vi "Parse Version String.vi"(11 "Version String":string) -> (3 "Version":T1)   [LabVIEW 2021, in "CIFPluginManager.lvclass"]
uses:
  CIFCore/Common/Typedef/Version.ctl
  <vilib>/regexp/Match Regular Expression.xnode
  CIFPluginManager.lvclass
  CIFPluginManager.lvclass/CIFPluginManager.ctl
  CIFCore/Common/CIFCoreCommon.lvlib
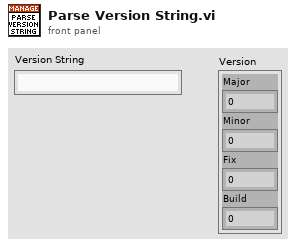
[diagram p1: front panel]
types:
  T1 = typedef "CIFCoreCommon.lvlib/Version.ctl" = cluster{"Major":i32, "Minor":i32, "Fix":i32, "Build":i32}
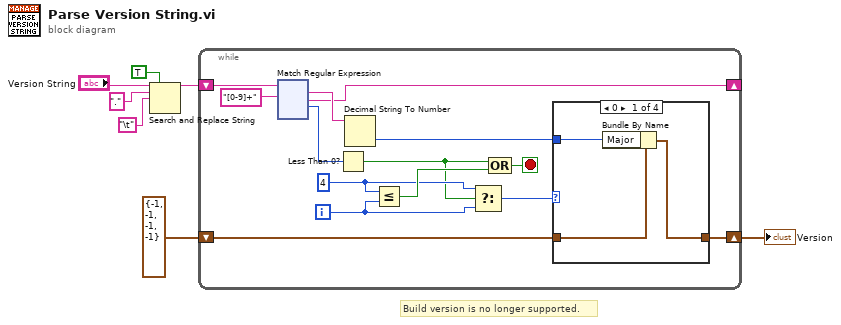
[diagram p0: block diagram]
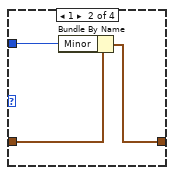
[diagram p2: hidden frame]
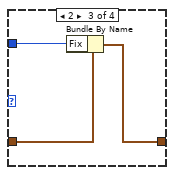
[diagram p3: hidden frame]
diagram:
  # "Build version is no longer supported."
  n1 = Search and Replace String(replace all?=TRUE ("replace all? (F)"), input string="Version String", search string=".", replace string="\t") -> (result string=w1:string)  [unwired: 4 in, 3 out]
  n2 = while {
    shift-right: [w20] -> w2
    shift-left: T1 {"Major"=-1, "Minor"=-1, "Fix"=-1, "Build"=-1} ("Version") -> [w21]
    shift-right: [w13] -> _
    shift-left: w1 -> [w15]
    i -> [w11]
    stop <- w18 stop-if-true
    w9 = 4 ("x")
    n3 = xnode "Match Regular Expression"("input string"=w15, "regular expression"="[0-9]+") -> ("whole match"=w14:string, "after match"=w13:string, "offset past match"=w12:i32)  [unwired: 4 in, 2 out]
    n4 = Less Than 0?(x=w12) -> (x < 0?=w8:bool)
    n5 = Decimal String To Number(string=w14) -> (number=w17:i32)  [unwired: 2 in, 1 out]
    n6 = Less Or Equal?(x=w9, y=w11) -> (x <= y?=w19:bool)
    n7 = Select(t=w9, s=w8, f=w11) -> (s? t:f=w10:i32)
    n8 = Compound Arithmetic op=OR(w8, w19) -> (w18:bool)
    n9 = case shown="0" w10 {
      tunnel: w17 -> [w140 w143 w146 _]
      tunnel: w21 -> [w141 w144 w147 w148]
      tunnel: [w139 w142 w145 w148] -> w20
      frame 0 {
        n10 = Bundle By Name(cluster=w141, "Major"=w140) -> (w139:T1)
      }
      frame 1 {
        n11 = Bundle By Name(cluster=w144, "Minor"=w143) -> (w142:T1)
      }
      frame 2 {
        n12 = Bundle By Name(cluster=w147, "Fix"=w146) -> (w145:T1)
      }
      frame 4, Default {
      }
    }
  }
  "Version" <- w2
